vi "readAutonCSV.vi"(2 "AutonFile":string) -> (6 "AutonArray":dbl[][](array[numeric]))   [LabVIEW 2012]
doc: "Use this VI to read comma delimited text files for input of autonomous data. Data should be in rows, in the following order: 1) Primitive ID number, 2) Heading (deg), 3) time(s)/Dist(in), 4) Power."
uses:
  <vilib>/Utility/file.llb/Read From Spreadsheet File (DBL).vi
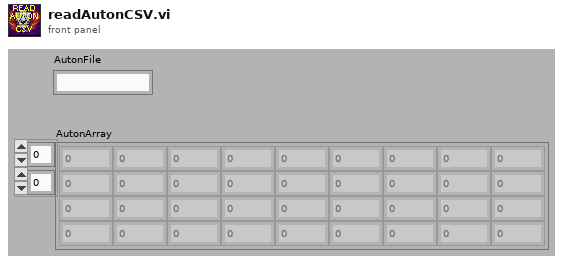
[diagram p1: front panel]
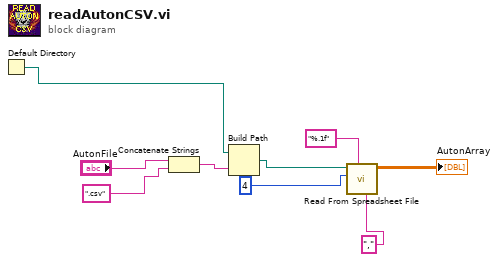
[diagram p0: block diagram]
diagram:
  n1 = Default Directory() -> (w4:path)
  n2 = Concatenate Strings("AutonFile", ".csv" ("string")) -> (w5:string)
  n3 = Build Path(base path=w4, name or relative path=w5) -> (appended path=w3:path)
  n4 = call-poly <vilib>:"Read From Spreadsheet File.vi"("delimiter (\\t)"="," ("delimiter (\\t)"), "format (%.3f)"="%.1f", "number of rows (all:-1)"=4, "file path (dialog if empty)"=w3) -> ("all rows"=→"AutonArray":dbl[][])  [unwired: 1 in, 6 out]
